vi "MT Calculate Worst Case Scaling Factor (Modulation and Resample).vi"   [LabVIEW 2020, in "niDMT.lvlib"]
doc: "Calculates the maximum possible peak amplitude, after pulse-shape filtering and resampling, of a waveform. This calculation is based on system parameters for a given modulation scheme."
uses:
  <vilib>/addons/Modulation/niDMT.lvlib
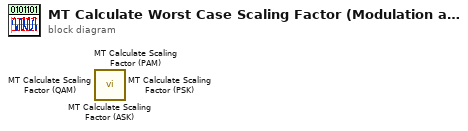
[diagram p0: block diagram]
diagram:
  n1 = call <vilib>:"MT Calculate Scaling Factor (ASK).vi"() -> ()  [unwired: 14 in, 2 out]
  n2 = call <vilib>:"MT Calculate Scaling Factor (PAM).vi"() -> ()  [unwired: 14 in, 2 out]
  n3 = call <vilib>:"MT Calculate Scaling Factor (QAM).vi"() -> ()  [unwired: 14 in, 2 out]
  n4 = call <vilib>:"MT Calculate Scaling Factor (PSK).vi"() -> ()  [unwired: 14 in, 2 out]
